vi "Add To Collection.vi"(8 "error in (no error)":errorcluster, 9 "IDrawable":refnum<class "IDrawable.lvclass">, 11 "Collection in":refnum<class "Collection.lvclass">) -> (0 "error out":errorcluster, 3 "Collection out":refnum<class "Collection.lvclass">)   [LabVIEW 2021, in "Picture2D.lvlib" / "Collection.lvclass"]
uses:
  Collection.lvclass
  IDrawable/IDrawable.lvclass
  Collection.lvclass/Collection.ctl
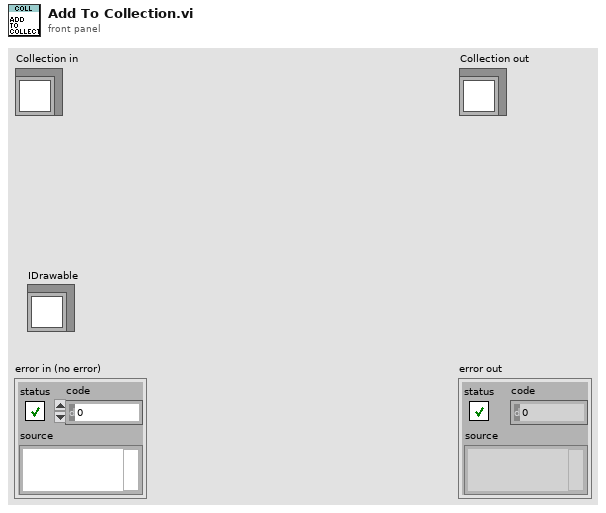
[diagram p1: front panel]
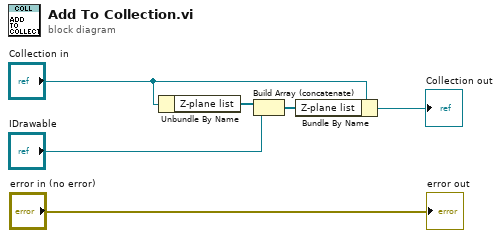
[diagram p0: block diagram]
diagram:
  n1 = Unbundle By Name("Collection in") -> ("Z-plane list"=w2:refnum<class "IDrawable.lvclass">[])
  n2 = Build Array (concatenate)(w2, "IDrawable") -> (w1:refnum<class "IDrawable.lvclass">[])
  n3 = Bundle By Name(cluster="Collection in", "Z-plane list"=w1) -> (→"Collection out":refnum<class "Collection.lvclass">)
  "error out" <- "error in (no error)"
